vi "Read JSON Config.vi"(8 "error in (no error)":errorcluster, 10 "JSON Config":string, 11 "Const_I8 in":refnum<class "Const_U8_1D.lvclass">) -> (0 "error out":errorcluster, 3 "Const_I8 out":refnum<class "Const_U8_1D.lvclass">)   [LabVIEW 2021, in "Const_U8_1D.lvclass"]
uses:
  Const_U8_1D.lvclass
  C:/Program Files (x86)/National Instruments/LabVIEW 2021/vi.lib/TSA/Abstract Data Classes/Abs_Types/Type/Abs_Type.lvclass
  Const_U8_1D.lvclass/Const_U8_1D.ctl
  22d55d5d-c6c8-4a9f-bf4e-773a84f34f3b.vi
  <vilib>/JDP Science/JSONtext/Find Item.vi
  <vilib>/JDP Science/JSONtext/Next JSON Value.vi
  <vilib>/JDP Science/JSONtext/String Subset.vi
  <vilib>/JDP Science/JSONtext/Parsing/Advance past next JSON Value (inlined COPY).vi
  <vilib>/JDP Science/JSONtext/Parsing/Advance past whitespace.vi
  <vilib>/JDP Science/JSONtext/Parsing/Advance past String.vi
  <vilib>/JDP Science/JSONtext/Parsing/Advance past Number.vi
  <vilib>/JDP Science/JSONtext/Parsing/Advance past Line Ending.vi
  <vilib>/Utility/LVClass/Get LV Class Name.vi
  <vilib>/JDP Science/JSONtext/Parsing/Parse Full Path or Item Name.vi
  <vilib>/JDP Science/JSONtext/Parsing/Advance past Array.vi
  <vilib>/JDP Science/JSONtext/Parsing/Advance past Object.vi
  <vilib>/JDP Science/JSONtext/support/Error Cluster From Code.vi
  <vilib>/JDP Science/JSONtext/Offset/Find Item Locations by Path.vi
  <vilib>/JDP Science/JSONtext/JSON text to Variant.vi
  <vilib>/JDP Science/JSONtext/LVClass Serializer/JSONtext LVClass Serializer.lvclass
  Abs_Types/U8 Integer 1D/Abs_U8 Integer 1D.lvclass
  Abs_Types/Type/Abs_Type.lvclass
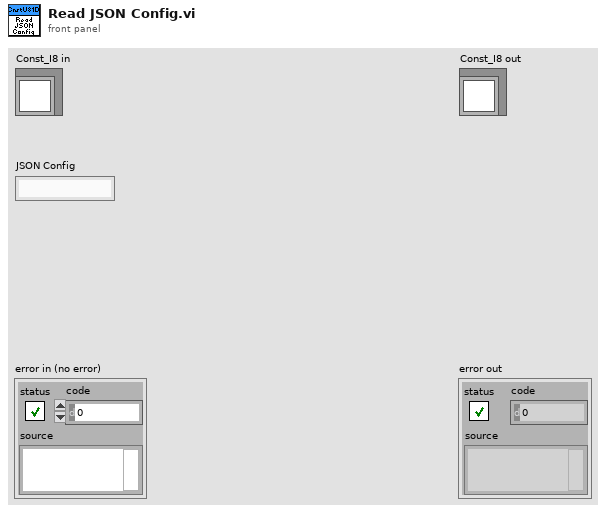
[diagram p1: front panel]
types:
  T1 = typedef "Const_U8_1D.lvclass/Type.ctl" = u8[]
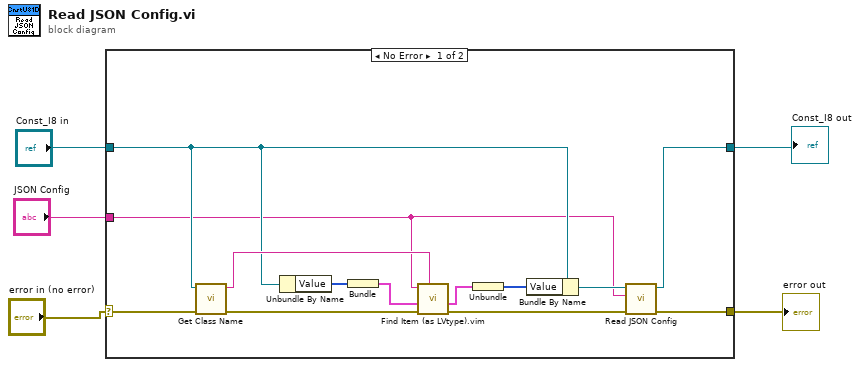
[diagram p0: block diagram]
diagram:
  n1 = case shown="No Error" "error in (no error)" {
    selector: "error in (no error)" -> [w11 w19]
    tunnel: [w18 w19] -> w3
    tunnel: [w17 w20] -> w4
    tunnel: "JSON Config" -> [w6 _]
    tunnel: "Const_I8 in" -> [w8 w20]
    frame No Error {
      n2 = call "Get Class Name.vi"("error in (no error)"=w11, "Abs_Type in"=w8) -> ("error out"=w9:errorcluster, "class name"=w10:string)  [unwired: 8 in]
      n3 = Unbundle By Name(w8) -> ("Value"=w12:T1)
      n4 = Bundle("Value"=w12) -> (w14:cluster{"Value":T1})  [unwired: 1 in]
      n5 = call "Find Item (as LVtype).vim"("$Path or Item Name"=w10, "error in (no error)"=w9, "Data Type and Default Value"=w14, "JSON"=w6) -> ("error out"=w13:errorcluster, "Data"=w15:cluster{"Value":T1})  [unwired: 4 in, 2 out]
      n6 = Unbundle(w15) -> ("Value"=w16:T1)
      n7 = Bundle By Name(cluster=w8, "Value"=w16) -> (w7:refnum<class "Const_U8_1D.lvclass">)
      n8 = call-parent "Read JSON Config.vi"("error in (no error)"=w13, "JSON Config"=w6, "Abs_Type in"=w7) -> ("error out"=w18:errorcluster, "Abs_Type out"=w17:refnum<class "Const_U8_1D.lvclass">)  [unwired: 7 in]
    }
    frame Error {
    }
  }
  "error out" <- w3
  "Const_I8 out" <- w4
